vi "getSerializedData.vi"(0 "reference":refnum<class "SystemNode.lvclass">, 5 "error in (no error)":errorcluster) -> (14 "reference out":refnum<class "SystemNode.lvclass">, 15 "parent":refnum<class "AbstractNode.lvclass">, 16 "children":refnum<class "AbstractNode.lvclass">[](array[class]), 17 "xmlOut":string, 19 "error out":errorcluster)   [LabVIEW 2020, in "SystemNode.lvclass"]
doc: "getSerializedData"
uses:
  <resource>/Framework/Providers/Open_GDS/UML/SystemNode_class/SystemNode.lvclass
  C:/Program Files (x86)/National Instruments/LabVIEW 2020/resource/Framework/Providers/Open_GDS/UML/RectangularNode_class/RectangularNode.lvclass
  C:/Program Files (x86)/National Instruments/LabVIEW 2020/resource/Framework/Providers/Open_GDS/UML/AbstractNode_class/AbstractNode.lvclass
  <resource>/Framework/Providers/Open_GDS/UML/AbstractNode_class/AbstractNode.lvclass
  <resource>/Framework/Providers/Open_GDS/UML/General/Rectangle/Rectangle Rectangle2D.ctl
  <resource>/Framework/Providers/Open_GDS/UML/MultiLineString_class/MultiLineString.lvclass
  <resource>/Framework/Providers/Open_GDS/UML/RectangularNode_class/RectangularNode.lvclass
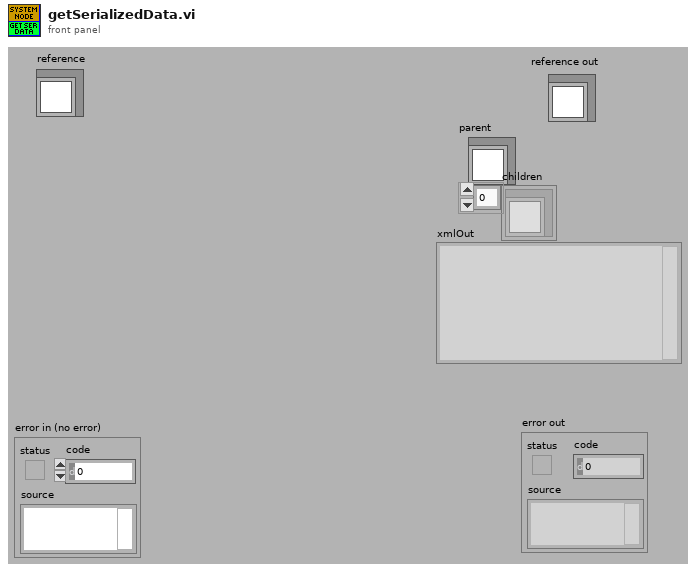
[diagram p1: front panel]
types:
  T1 = typedef "Rectangle Rectangle2D.ctl" = cluster{"x":dbl, "y":dbl, "width":dbl, "height":dbl}
  T2 = cluster{"Base class":cluster{"Base class":cluster{"parent":refnum<k1>, "children":refnum<k1>[]}, "bounds":T1}, "contents":refnum<k1>, "DEFAULT_WIDTH":i32, "DEFAULT_HEIGHT":i32, "NAME_GAP":i32, "XGAP":i32, "YGAP":i32}
  T3 = typedef "SystemNode.lvclass/ObjectAttributes.ctl" = cluster{"contents":refnum<class "MultiLineString.lvclass">, "DEFAULT_WIDTH":i32, "DEFAULT_HEIGHT":i32, "NAME_GAP":i32, "XGAP":i32, "YGAP":i32}
  T4 = typedef "RectangularNode.lvclass/ObjectAttributes.ctl" = cluster{"bounds":T1}
  T5 = typedef "AbstractNode.lvclass/ObjectAttributes.ctl" = cluster{"parent":refnum<class "AbstractNode.lvclass">, "children":refnum<class "AbstractNode.lvclass">[], "Hidden":bool}
  T6 = cluster{"Attributes":cluster{"Base class":cluster{"Base class":cluster{"parent":refnum<k1>, "children":refnum<k1>[]}, "bounds":T1}, "contents":refnum<k1>, "DEFAULT_WIDTH":i32, "DEFAULT_HEIGHT":i32, "NAME_GAP":i32, "XGAP":i32, "YGAP":i32}, "text":string}
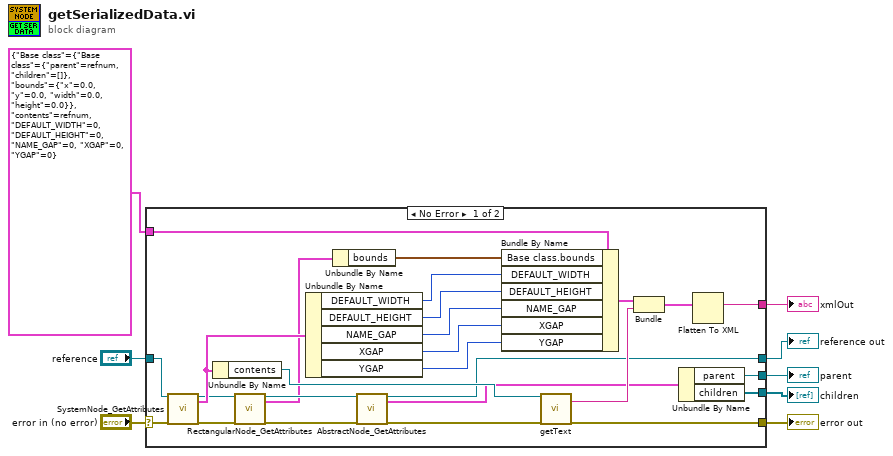
[diagram p0: block diagram]
diagram:
  n1 = case shown="No Error" "error in (no error)" {
    selector: "error in (no error)" -> [w34 w35]
    tunnel: "reference" -> [w33 w36]
    tunnel: [w29 w35] -> w6
    tunnel: [w11 w36] -> w5
    tunnel: [w28 _] -> w4
    tunnel: [w27 _] -> w3
    tunnel: [w26 _] -> w2
    tunnel: T2 {"Base class"={"Base class"={"parent"=refnum, "children"=[]}, "bounds"={"x"=0.0, "y"=0.0, "width"=0.0, "height"=0.0}}, "contents"=refnum, "DEFAULT_WIDTH"=0, "DEFAULT_HEIGHT"=0, "NAME_GAP"=0, "XGAP"=0, "YGAP"=0} ("Attributes") -> [w25 _]
    frame No Error {
      n2 = call <resource>:"SystemNode_GetAttributes.vi"("reference in"=w33, "error in (no error)"=w34) -> ("reference out"=w16:refnum<class "SystemNode.lvclass">, "Data"=w17:T3, "error out"=w15:errorcluster)  [unwired: 1 in, 14 out]
      n3 = Unbundle By Name(w17) -> ("contents"=w30:refnum<class "MultiLineString.lvclass">)
      n4 = call <resource>:"RectangularNode_GetAttributes.vi"("reference in"=w16, "error in (no error)"=w15) -> ("reference out"=w14:refnum<class "SystemNode.lvclass">, "Data"=w10:T4, "error out"=w13:errorcluster)  [unwired: 14 in, 1 out]
      n5 = Unbundle By Name(w17) -> ("DEFAULT_WIDTH"=w22:i32, "DEFAULT_HEIGHT"=w21:i32, "NAME_GAP"=w20:i32, "XGAP"=w19:i32, "YGAP"=w18:i32)
      n6 = Unbundle By Name(w10) -> ("bounds"=w23:T1)
      n7 = call <resource>:"AbstractNode_GetAttributes.vi"("reference in"=w14, "error in (no error)"=w13) -> ("reference out"=w11:refnum<class "SystemNode.lvclass">, "Data"=w9:T5, "error out"=w12:errorcluster)  [unwired: 14 in, 1 out]
      n8 = Bundle By Name(cluster=w25, "Base class.bounds"=w23, "DEFAULT_WIDTH"=w22, "DEFAULT_HEIGHT"=w21, "NAME_GAP"=w20, "XGAP"=w19, "YGAP"=w18) -> (w24:T2)
      n9 = call-dynamic "getText.vi"("reference"=w30, "error in (no error)"=w12) -> ("text"=w31:string, "error out"=w29:errorcluster)  [unwired: 16 out]
      n10 = Bundle("Attributes"=w24, "text"=w31) -> (w32:T6)  [unwired: 1 out]
      n11 = Unbundle By Name(w9) -> ("parent"=w28:refnum<class "AbstractNode.lvclass">, "children"=w27:refnum<class "AbstractNode.lvclass">[])
      n12 = Flatten To XML(6:w32) -> (2:w26:string)
    }
    frame Error {
    }
  }
  "reference out" <- w5
  "error out" <- w6
  "parent" <- w4
  "children" <- w3
  "xmlOut" <- w2
